vi "client.vi"() -> ()   [LabVIEW 2020]
uses:
  Global_Variable/Global.vi
panel:
  in  "设备信息":T1
  in  "服务器关闭":string="服务器VI关闭了连接。"
  in  "停止":bool
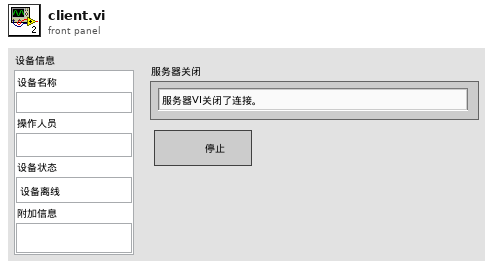
[diagram p1: front panel]
types:
  T1 = cluster{"设备名称":string, "操作人员":string, "设备状态":enum16{"设备离线", "设备正常", "设备缺料", "设备故障", "质量报警"}, "附加信息":string}
  T2 = enum32{"Invalid", "Standard", "Closed", "Hidden", "Minimized", "Maximized"}
  T3 = cluster{"设备名称":bool, "操作人员":bool, "设备状态":bool, "附加信息":bool}
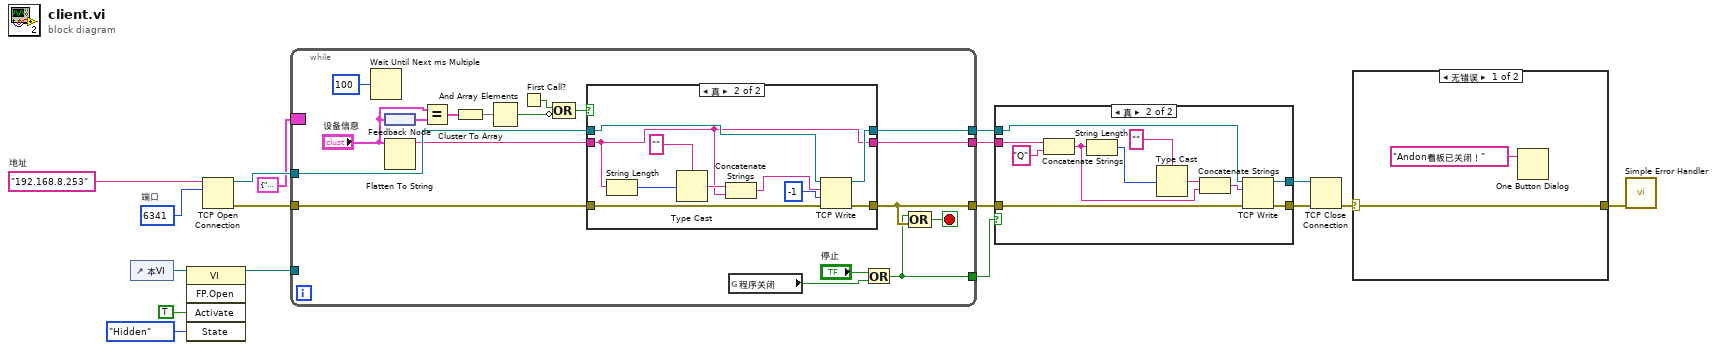
[diagram p0: block diagram]
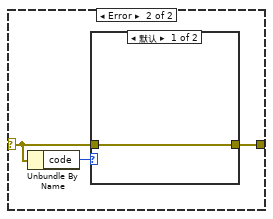
[diagram p2: hidden frame]
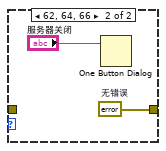
[diagram p3: hidden frame]
diagram:
  w1 = "192.168.8.253"  # 地址
  w17 = u16 6341  # 端口
  n1 = control-ref of="本VI"() -> (w3:refnum<vi>)
  n2 = invoke class="VI" method="FP.Open"(reference=w3, "Activate"=TRUE ("激活？"), "State"=T2."Hidden" ("状态")) -> (reference out=w2:refnum<vi>)  [unwired: 2 in, 4 out]
  n3 = TCP Open Connection(address=w1, remote port or service name=w17) -> (connection ID=w16:refnum<k5>, error out=w15:errorcluster)  [unwired: 1 in, 2 out]
  n4 = while {
    tunnel: [w22] -> w10
    tunnel: [w33] -> w14
    tunnel: [w30] -> w12
    tunnel: w15 -> [w34]
    tunnel: w16 -> [w35]
    tunnel: [w23] -> w7
    border: T1 {"设备名称"="", "操作人员"="", "设备状态"=enum."设备正常", "附加信息"=""} ("设备信息") -> [_]
    tunnel: w2 -> [_]
    stop <- w32 stop-if-true
    n5 = Wait Until Next ms Multiple(millisecond multiple=u32 100 ("毫秒倍数")) -> ()  [unwired: 1 out]
    n6 = feedback-in #1("设备信息") -> ()
    n7 = feedback #1() -> (w27:T1)
    n8 = Flatten To String(anything="设备信息") -> (data string=w24:string)  [unwired: 3 in, 2 out]
    n9 = Equal?(x="设备信息", y=w27) -> (x = y?=w26:T3)
    n10 = Cluster To Array(cluster=w26) -> (array=w25:bool[])
    n11 = And Array Elements(Boolean array=w25) -> (logical AND=w18:bool)
    n12 = First Call?() -> (First Call?: T/F=w20:bool)
    n13 = Compound Arithmetic op=OR ("复合运算")(w20, invert w18) -> (w19:bool)
    n14 = case shown="真" w19 {
      tunnel: w35 -> [w38 w48]
      tunnel: w34 -> [w37 w47]
      tunnel: [w38 w46] -> w33
      tunnel: [w37 w45] -> w30
      tunnel: w24 -> [w36 w39]
      tunnel: [w36 w39] -> w23
      frame False {
      }
      frame True {
        n15 = String Length(string=w39) -> (length=w43:i32)
        n16 = Type Cast(type="", x=w43) -> (*(type *) &x=w41:string)
        n17 = Concatenate Strings(w41, w39) -> (w40:string)
        n18 = TCP Write(connection ID=w48, data in=w40, error in (no error)=w47, 9:-1) -> (connection ID out=w46:refnum<k5>, error out=w45:errorcluster)  [unwired: 1 out]
      }
    }
    n19 = global read "Global.vi" "程序关闭"() -> (w21:bool)
    n20 = Or(x="停止", y=w21) -> (x .or. y?=w22:bool)
    n21 = Compound Arithmetic op=OR ("复合运算")(w22, w30) -> (w32:bool)
  }
  n22 = case shown="真" w10 {
    tunnel: w14 -> [w50 w61]
    tunnel: [w50 w59] -> w13
    tunnel: w12 -> [w49 w60]
    tunnel: [w49 w58] -> w11
    tunnel: w7 -> [_ w56]
    frame False {
    }
    frame True {
      n23 = Concatenate Strings(w56, "Q") -> (w52:string)
      n24 = String Length(string=w52) -> (length=w55:i32)
      n25 = Type Cast(type="", x=w55) -> (*(type *) &x=w53:string)
      n26 = Concatenate Strings(w53, w52) -> (w51:string)
      n27 = TCP Write(connection ID=w61, data in=w51, error in (no error)=w60) -> (connection ID out=w59:refnum<k5>, error out=w58:errorcluster)  [unwired: 2 out]
    }
  }
  n28 = TCP Close Connection(connection ID=w13, error in (no error)=w11) -> (error out=w9:errorcluster)  [unwired: 2 out]
  n29 = case shown="无错误" w9 {
    selector: w9 -> [w63 w65]
    tunnel: [w63 w64] -> w8
    frame No Error {
      n30 = One Button Dialog(message="Andon看板已关闭！" ("消息")) -> ()  [unwired: 1 in, 1 out]
    }
    frame Error {
      n31 = Unbundle By Name(w65) -> ("code"=w66:i32)
      n32 = case shown="默认" w66 {
        tunnel: w65 -> [w67 _]
        tunnel: [w67 w69] -> w64
        frame Default {
        }
        frame 62, 64, 66 {
          w69 = errorcluster {"status"=FALSE, "code"=0, "source"=""}  # 无错误
          n33 = One Button Dialog(message="服务器关闭") -> ()  [unwired: 1 in, 1 out]
        }
      }
    }
  }
  n34 = call <vilib>:"Simple Error Handler.vi"("error in (no error)"=w8) -> ()  [unwired: 1 in, 8 out]
